vi "getWidthAndHight.vi"(1 "OldBnds":T1) -> (0 "output cluster":cluster{"X":sgl, "Y":sgl})   [LabVIEW 2013]
uses:
  <vilib>/Utility/miscctls.llb/LVRectTypeDef.ctl
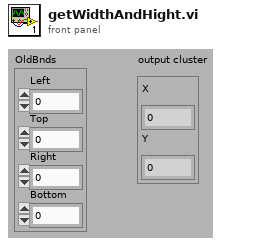
[diagram p1: front panel]
types:
  T1 = typedef "LVRectTypeDef.ctl" = cluster{"Left":i16, "Top":i16, "Right":i16, "Bottom":i16}
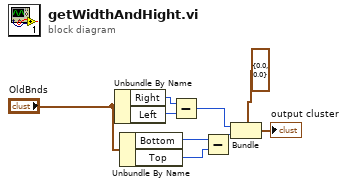
[diagram p0: block diagram]
diagram:
  n1 = Unbundle By Name("OldBnds") -> ("Right"=w7:i16, "Left"=w8:i16)
  n2 = Unbundle By Name("OldBnds") -> ("Bottom"=w3:i16, "Top"=w4:i16)
  n3 = Subtract(x=w7, y=w8) -> (x-y=w1:i16)
  n4 = Subtract(x=w3, y=w4) -> (x-y=w6:i16)
  n5 = Bundle(cluster=cluster{"X":sgl, "Y":sgl} {"X"=0.0, "Y"=0.0} ("ZoomSingle:All Elements"), "X"=w1, "Y"=w6) -> (→"output cluster":cluster{"X":sgl, "Y":sgl})
